vi "status.vi"(3 "error in (no error)":errorcluster, 5 "HGF_DSCMonitor":refnum<class "HGF_DSCMonitor.lvclass">) -> (0 "error out":errorcluster, 1 "Array":T1(array[cluster]), 2 "dup HGF_DSCMonitor":refnum<class "HGF_DSCMonitor.lvclass">)   [LabVIEW 2012, in "HGF_DSC.lvlib" / "HGF_DSCMonitor.lvclass"]
doc: "Request status from monitor"
uses:
  HGF_DSCMonitor.lvclass
  HGF_BaseClasses/HGF_NetworkVisitor/HGF_NetworkVisitor.lvclass
  HGF_BaseClasses/HGF_TriggeredEvent/HGF_TriggeredEvent.lvclass
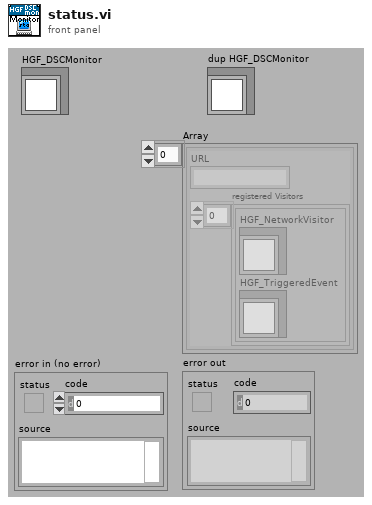
[diagram p1: front panel]
types:
  T1 = cluster{"URL":string, "registered Visitors":cluster{"HGF_NetworkVisitor":refnum<class "HGF_NetworkVisitor.lvclass">, "HGF_TriggeredEvent":refnum<class "HGF_TriggeredEvent.lvclass">}[]}[]
  T2 = cluster{"Shared Variable":refnum<k21>, "registered Visitors":cluster{"HGF_NetworkVisitor":refnum<class "HGF_NetworkVisitor.lvclass">, "HGF_TriggeredEvent":refnum<class "HGF_TriggeredEvent.lvclass">}[]}[]
  T3 = cluster{"HGF_NetworkVisitor":refnum<class "HGF_NetworkVisitor.lvclass">, "HGF_TriggeredEvent":refnum<class "HGF_TriggeredEvent.lvclass">}[]
  T4 = cluster{string, "registered Visitors":cluster{"HGF_NetworkVisitor":refnum<class "HGF_NetworkVisitor.lvclass">, "HGF_TriggeredEvent":refnum<class "HGF_TriggeredEvent.lvclass">}[]}
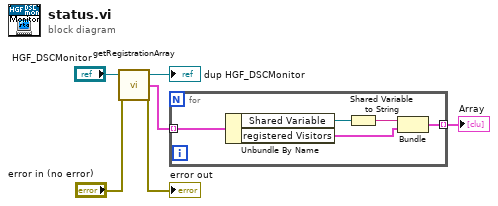
[diagram p0: block diagram]
diagram:
  n1 = call "getRegistrationArray.vi"("error in (no error)"="error in (no error)", "HGF_DSCMonitor"="HGF_DSCMonitor") -> ("error out"=→"error out":errorcluster, "Registration Array"=w2:T2, "HGF_DSCMonitor"=→"dup HGF_DSCMonitor":refnum<class "HGF_DSCMonitor.lvclass">)  [unwired: 1 in]
  n2 = for {
    tunnel: w2 -> [w11] mode=indexing
    tunnel: [w7] -> w1 mode=indexing
    n3 = Unbundle By Name(w11) -> ("Shared Variable"=w9:refnum<k21>, "registered Visitors"=w10:T3)
    n4 = Shared Variable to String(1:w9) -> (0:w8:string)
    n5 = Bundle(w8, "registered Visitors"=w10) -> (w7:T4)  [unwired: 1 in]
  }
  "Array" <- w1
